vi "Create DaqLoopTimer Q.vi"(8 "error in (no error)":errorcluster, 11 "QName":string) -> (0 "error out":errorcluster, 3 "DaqData ElapsedTimeRef":refnum<queue>)   [LabVIEW 2017, in "DAQ.lvclass"]
doc: "Developed by Kevin Thompson\nThompson Engineering, LLC\nkevin@thompsonengineering.net"
uses:
  DAQ.lvclass
  GBL DataQ Refs.vi
panel:
  out "data reference":u32
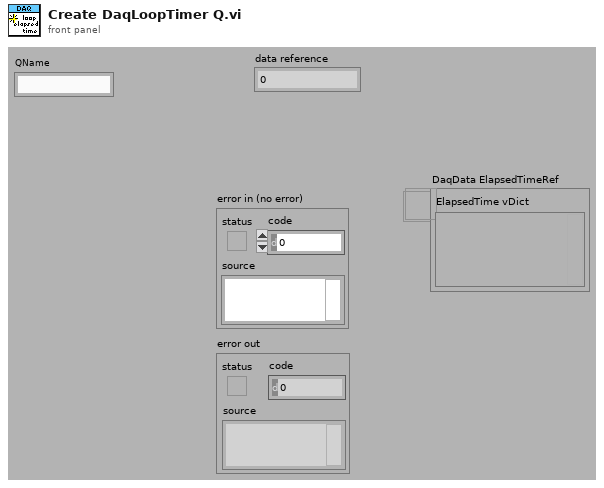
[diagram p1: front panel]
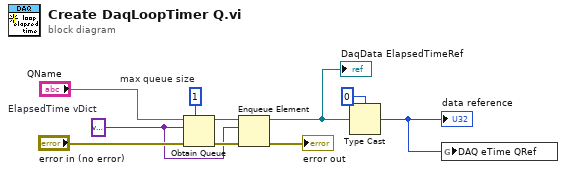
[diagram p0: block diagram]
diagram:
  w1 = variant  # ElapsedTime vDict
  w9 = 1  # max queue size
  n1 = Obtain Queue(max queue size (-1, unlimited)=w9, name (unnamed)="QName", element data type=w1, error in (no error)="error in (no error)") -> (queue out=w7:refnum<queue>, error out=w8:errorcluster)  [unwired: 1 in, 1 out]
  n2 = Enqueue Element(queue=w7, element=w1, error in (no error)=w8) -> (queue out=w4:refnum<queue>, error out=→"error out":errorcluster)  [unwired: 1 in, 1 out]
  "DaqData ElapsedTimeRef" <- w4
  n3 = Type Cast(type=u32 0, x=w4) -> (*(type *) &x=w2:u32)
  "data reference" <- w2
  n4 = global write "GBL DataQ Refs.vi" "DAQ eTime QRef"(w2) -> ()
